vi "View TDMS Content.vi"() -> ()   [LabVIEW 2019]
uses:
  <vilib>/Utility/Data Type/Type Definitions/Type Definition Info.ctl
  <vilib>/Utility/Data Type/Type Definitions/Data Type.ctl
  <vilib>/Utility/Data Type/NI_Data Type.lvlib
panel:
  out "Values":string[](array[string])
  out "Name":string[](array[string])
  out "Type":T1[](array[typedef])
  out "Type def info":T2[](array[typedef])
  out "property values":variant[](array[variant])
  out "property names":string[](array[string])
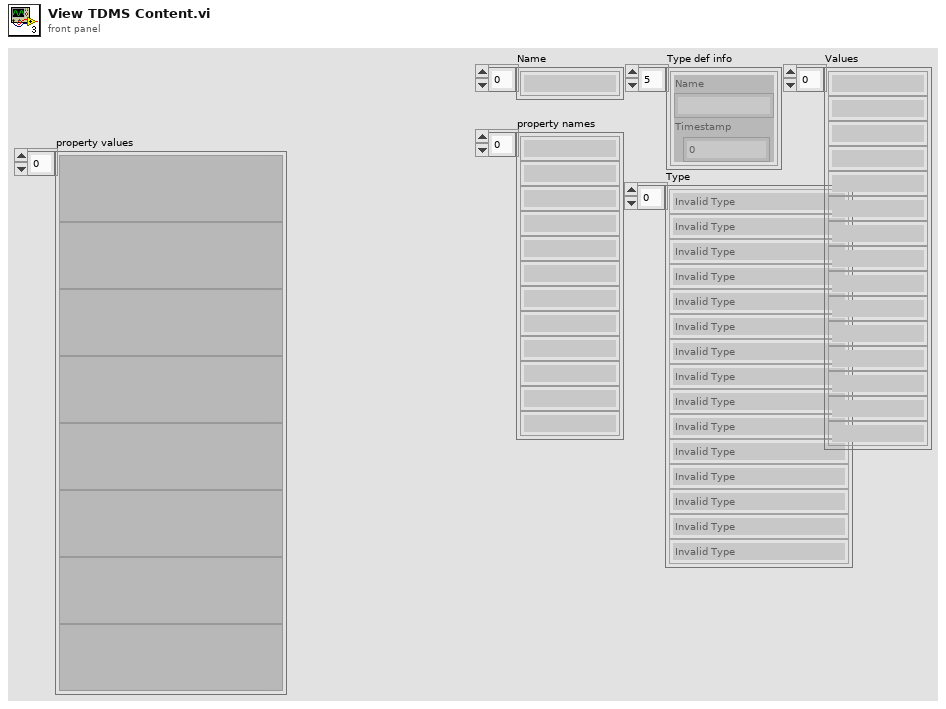
[diagram p1: front panel]
types:
  T1 = typedef "NI_Data Type.lvlib/Data Type.ctl" = enum8{"Invalid Type", "Void", "I8", "I16", "I32", "I64", "U8", "U16", "U32", "U64", "Single Float", "Double Float", "Extended Float", "Single Complex", "Double Complex", "Extended Complex", "Enum U8", "Enum U16", "Enum U32", "Enum U64", "Single Float With Unit", "Double Float With Unit", "Extended Float With Unit", "Single Complex with Unit", "Double Complex with Unit", "Extended Complex with Unit", "Boolean", "String", "Path", "Picture", "Tag", "Array", "Cluster", "Variant", "LV Variant", "Waveform", "Timestamp", "Digital Waveform", "Digital Data", "ExpressData", "Refnum", "External Data", "VI", "Poly VI", "LabVIEW Class Instance", "Fixed Point", "Set Collection", "Map Collection"}
  T2 = typedef "NI_Data Type.lvlib/Type Definition Info.ctl" = cluster{"Name":string, "Timestamp":u32}
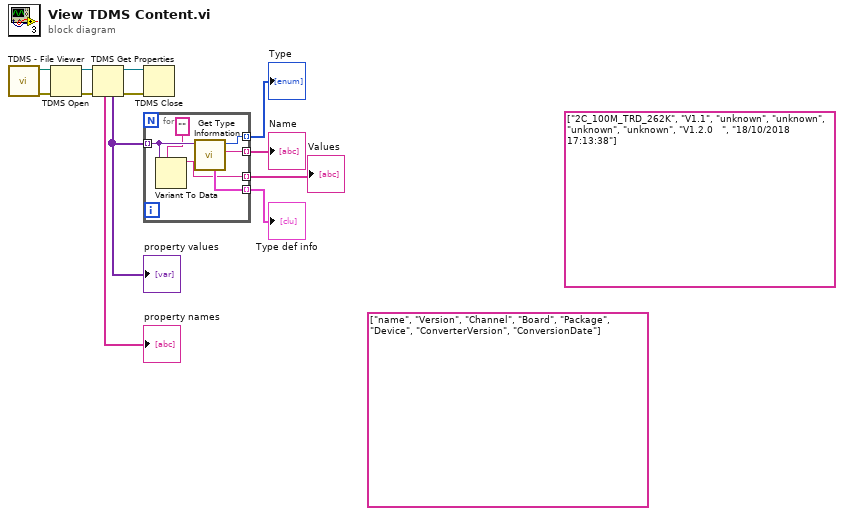
[diagram p0: block diagram]
diagram:
  (unwired) string[] ["name", "Version", "Channel", "Board", "Package", "Device", "ConverterVersion", "ConversionDate"] ("property names")
  (unwired) string[] ["2C_100M_TRD_262K", "V1.1", "unknown", "unknown", "unknown", "unknown", "V1.2.0   ", "18/10/2018 17:13:38"] ("Values")
  n1 = call <vilib>:"TDMS - File Viewer.vi"() -> ("error out"=w11:errorcluster, "file path out"=w12:path)  [unwired: 6 in]
  n2 = TDMS Open(8:w11, 11:w12) -> (0:w9:errorcluster, 3:w10:refnum<k34>)  [unwired: 5 in]
  n3 = TDMS Get Properties(8:w9, 11:w10) -> (0:w7:errorcluster, 3:w8:refnum<k34>, 4:w5:variant[], 6:→"property names":string[])  [unwired: 4 in, 2 out]
  "property values" <- w5
  n4 = TDMS Close(8:w7, 11:w8) -> ()  [unwired: 2 out]
  n5 = for {
    tunnel: w5 -> [w15] mode=indexing
    tunnel: [w18] -> w3 mode=indexing
    tunnel: [w17] -> w4 mode=indexing
    tunnel: [w16] -> w2 mode=indexing
    tunnel: [w13] -> w1 mode=indexing
    n6 = Variant To Data(type="", Variant=w15) -> (data=w13:string)  [unwired: 1 in, 1 out]
    n7 = call <vilib>:"Get Type Information.vi"("variant"=w15) -> ("name"=w16:string, "type"=w18:T1, "type definition info"=w17:T2)  [unwired: 6 in, 2 out]
  }
  "Type def info" <- w4
  "Type" <- w3
  "Name" <- w2
  "Values" <- w1
